vi "Unregister Plugin.vi"(6 "timeout (ms)":i32=500, 8 "error in":errorcluster, 10 "Unregister":T1, 11 "gRPC ID in":T2) -> (0 "error out":errorcluster, 3 "gRPC ID out":T2)   [LabVIEW 2021, in "CIFManagerClientWrapper.lvlib"]
uses:
  CIFManagerClientWrapper.lvlib
  CIF_Manager_client/CIF_Manager_client.lvlib
  <vilib>/gRPC/LabVIEW gRPC Library/Shared/grpcId.ctl
  <vilib>/gRPC/LabVIEW gRPC Library/grpc-lvsupport-release.lvlib
  CIF_Manager_client/RPC Messages/cif_manager_UnregisterData.ctl
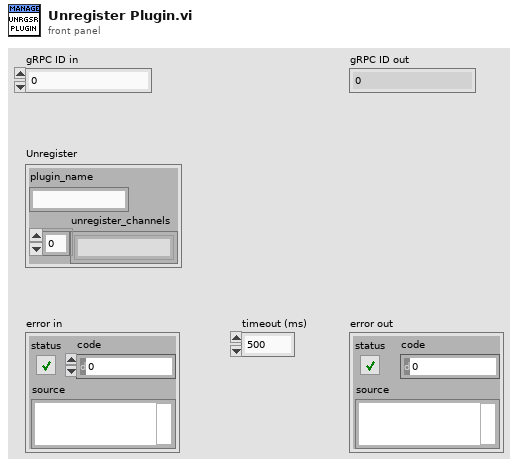
[diagram p1: front panel]
types:
  T1 = typedef "CIF_Manager_client.lvlib/cif_manager_UnregisterData.ctl" = cluster{"plugin_name":string, "unregister_channels":string[]}
  T2 = typedef "grpc-lvsupport-release.lvlib/grpcId.ctl" = u64
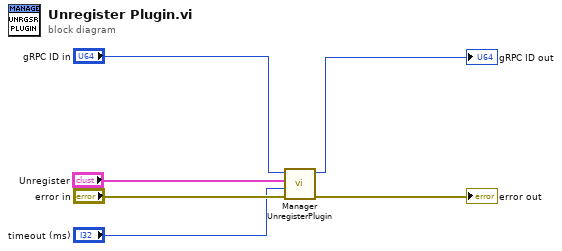
[diagram p0: block diagram]
diagram:
  n1 = call "Manager UnregisterPlugin.vi"("error in"="error in", "timeout (ms)"="timeout (ms)", "Request Data"="Unregister", "gRPC ID"="gRPC ID in") -> ("error out"=→"error out":errorcluster, "gRPC ID out"=→"gRPC ID out":T2)  [unwired: 5 in, 1 out]
